vi "spread_nan.vi"(6 "type":i32(ring) items=["standard deviation", "range", "mean absolute deviation", "interquartile range"], 7 "Array":dbl[](array[numeric])) -> (0 "error":i32, 3 "spread":dbl)   [LabVIEW 2016, in "nan operations.lvlib"]
uses:
  nan operations.lvlib
  <vilib>/gmath/NI_Gmath.lvlib
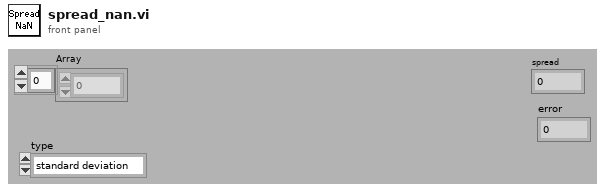
[diagram p1: front panel]
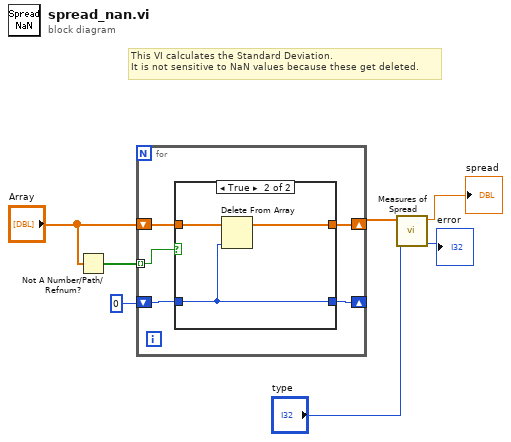
[diagram p0: block diagram]
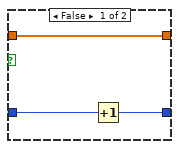
[diagram p2: hidden frame]
diagram:
  # "This VI calculates the Standard Deviation. \nIt is not sensitive to NaN values because these get deleted."
  n1 = Not A Number/Path/Refnum?(number/path/refnum="Array") -> (NaN/Path/Refnum?=w7:bool[])
  n2 = for {
    tunnel: w7 -> [w11] mode=indexing
    shift-right: [w10] -> w5
    shift-left: "Array" -> [w12]
    shift-right: [w9] -> _
    shift-left: 0 -> [w8]
    n3 = case shown="True" w11 {
      tunnel: w12 -> [w15 w18]
      tunnel: [w15 w17] -> w10
      tunnel: [w13 w16] -> w9
      tunnel: w8 -> [w14 w16]
      frame False {
        n4 = Increment(x=w14) -> (x+1=w13:i32)
      }
      frame True {
        n5 = Delete From Array(array=w18, index=w16) -> (array with subset deleted=w17:dbl[])  [unwired: 1 in, 1 out]
      }
    }
  }
  n6 = call <vilib>:"Measures of Spread.vi"("type"="type", "x array"=w5) -> ("error"=→"error":i32, "spread value"=→"spread":dbl)  [unwired: 8 in]
